vi "OverlayPoints_2D.vi"(6 "Color":u32(colorbox)=16711680, 7 "GroupName":string, 8 "error in":errorcluster, 10 "Points":T1[][](array[typedef]), 11 "Image Reference In":T2) -> (0 "error out":errorcluster, 3 "Image Reference Out":T2)   [LabVIEW 2020, in "OpenLvVision_Overlays.lvlib"]
doc: "Overlays a point on top of an image."
uses:
  OpenLvVision_Overlays.lvlib
  <vilib>/OpenLvVision/OpenLvVision_Image/Management/TypeDef/OLV Image.ctl
  <vilib>/OpenLvVision/OpenLvVision_Image/Management/OLV Management.lvlib
  TypeDefs/PointI32.ctl
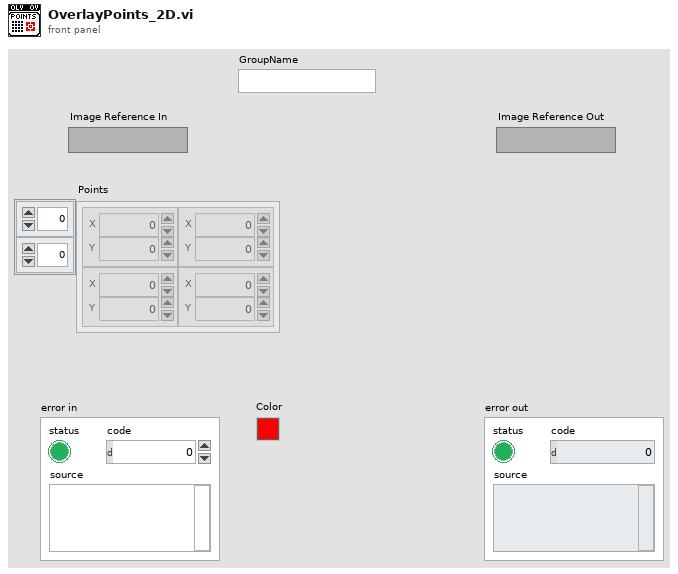
[diagram p1: front panel]
types:
  T1 = typedef "OpenLvVision_Overlays.lvlib/PointI32.ctl" = cluster{"X":i32, "Y":i32}
  T2 = typedef "OLV OpenLvVision_Image.lvlib/OLV Management.lvlib/OLV Image.ctl" = refnum<image>
  T3 = typedef "IMAQ Image.ctl" = refnum<image>
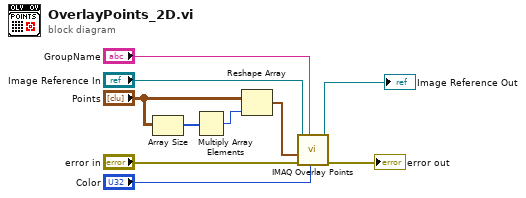
[diagram p0: block diagram]
diagram:
  n1 = Array Size(array="Points") -> (size(s)=w1:i32[])
  n2 = Multiply Array Elements(1:w1) -> (0:w2:i32)
  n3 = Reshape Array("Points", w2) -> (w4:T1[])
  n4 = call "IMAQ Overlay Points"("Color"="Color", "Group"="GroupName", "error in (no error)"="error in", "Array of Points"=w4, "Image"="Image Reference In") -> ("error out"=→"error out":errorcluster, "Image Out"=→"Image Reference Out":T3)  [unwired: 5 in]
